vi "huan+.vi"(8 "当前PWM":dbl=1.0, 9 "缓起清零":bool, 10 "循环数(100)":dbl=100.0, 11 "值":dbl) -> (3 "数值":dbl=1.0)   [LabVIEW 2017]
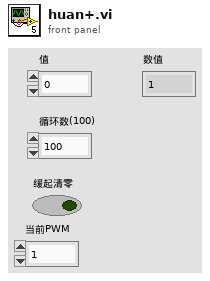
[diagram p1: front panel]
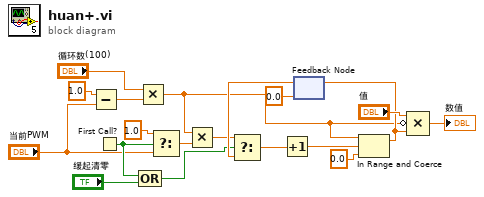
[diagram p0: block diagram]
diagram:
  n1 = Subtract(x=1.0, y="当前PWM") -> (x-y=w3:dbl)
  n2 = First Call?() -> (First Call?: T/F=w8:bool)
  n3 = Multiply(x="循环数(100)", y=w3) -> (x*y=w1:dbl)
  n4 = Compound Arithmetic op=OR ("复合运算")(w8, "缓起清零") -> (w13:bool)
  n5 = Select(t=1.0 ("f"), s=w8, f="当前PWM") -> (s? t:f=w9:dbl)
  n6 = Multiply(x=w1, y=w9) -> (x*y=w6:dbl)
  n7 = feedback #1(0.0) -> (w15:dbl)
  n8 = Select(t=w6, s=w13, f=w15) -> (s? t:f=w14:dbl)
  n9 = Increment(x=w14) -> (x+1=w11:dbl)
  n10 = In Range and Coerce(upper limit=w1, x=w11, lower limit=0.0 ("下限")) -> (coerced(x)=w10:dbl)  [unwired: 1 out]
  n11 = feedback-in #1(w10) -> ()
  n12 = Compound Arithmetic op=MULTIPLY("值", invert w1, w10) -> (→"数值":dbl)
